vi "AutoDrive_sub.vi"(10 "Drive Control":T2={"Left X"=0, "Left Y"=0, "Right X"=0, "Power (100)"=100, "Wait (ms)"=100} {"Power (100)" min=-100 max=100}, 11 "NXT/EV3":T1) -> (3 "NXT/EV3 out":T1)   [LabVIEW 2012, in "Mecanum Drive.lvrbt"]
uses:
  Mecanum Drive.lvrbt
  SubVIs/auto_drive_TYP.ctl
  <vilib>/NXT/Subs/LVHSConnector.ctl
  <vilib>/NXT/LegoClasses/BrickReference/BrickReference.lvclass
  <vilib>/FTC/FTC ControllerState.ctl
  <vilib>/FTC/FTC POVState.ctl
  <vilib>/NXT/Hardware/Plugins/Tetrix DC Motor/TetrixDCMotorAddress.ctl
  <vilib>/NXT/Dual Mode Library/Display/drawNumber.vi
  <vilib>/NXT/NXTIO Xnodes/NXTIONodeSubVIs/TETRIX IO Move DC Motors.vi
  <vilib>/NXT/Dual Mode Library/Waits/Wait_Num(msec).vi
  <vilib>/NXT/NXTIO Xnodes/AddressXNode/NXTIOAddress.xnode
  <vilib>/NXT/NXTIO Xnodes/NXTIOXNode/NXTIO.xnode
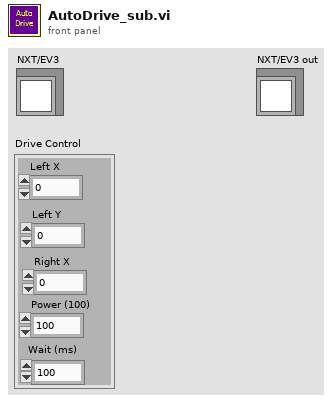
[diagram p1: front panel]
types:
  T1 = typedef "LVHSConnector.ctl" = refnum<class "BrickReference.lvclass">
  T2 = typedef "auto_drive_TYP.ctl" = cluster{"Left X":i8, "Left Y":i8, "Right X":i8, "Power (100)":i8, "Wait (ms)":u32}
  T3 = typedef "FTC ControllerState.ctl" = cluster{"Left X":i8, "Left Y":i8, "Right X":i8, "Right Y":i8, "Button Encoding 9-12":u8, "Button Encoding 1-8":u8, "POV":T4}
  T4 = typedef "FTC POVState.ctl" = i8
  T5 = typedef "TetrixDCMotorAddress.ctl" = i32
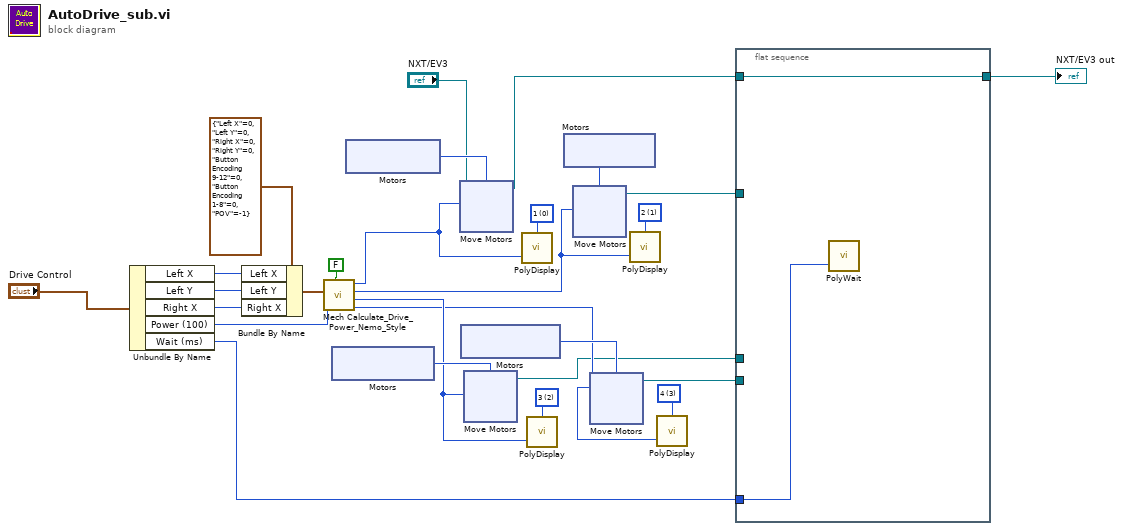
[diagram p0: block diagram]
diagram:
  w17 = i16 3 items=["1", "2", "3", "4", "5", "6", "7", "8", "9", "10", "11", "12"] ("Line")
  w19 = i16 2 items=["1", "2", "3", "4", "5", "6", "7", "8", "9", "10", "11", "12"] ("Line")
  w21 = i16 1 items=["1", "2", "3", "4", "5", "6", "7", "8", "9", "10", "11", "12"] ("Line")
  w22 = i16 0 items=["1", "2", "3", "4", "5", "6", "7", "8", "9", "10", "11", "12"] ("Line")
  n1 = Unbundle By Name("Drive Control") -> ("Left X"=w10:i8, "Left Y"=w9:i8, "Right X"=w8:i8, "Power (100)"=w2:i8, "Wait (ms)"=w1:u32)
  n2 = Bundle By Name(cluster=T3 {"Left X"=0, "Left Y"=0, "Right X"=0, "Right Y"=0, "Button Encoding 9-12"=0, "Button Encoding 1-8"=0, "POV"=-1} ("Controller State"), "Left X"=w10, "Left Y"=w9, "Right X"=w8) -> (w14:T3)
  n3 = call "Mech Calculate_Drive_Power_Nemo_Style.vi"("Reverse"=FALSE, "Controller State"=w14, "Power Level (100)"=w2) -> ("Right Rear Power"=w16:i8, "Right Front Power"=w18:i8, "Left Rear Power"=w20:i8, "Left Front Power"=w15:i8)  [unwired: 5 in]
  n4 = xnode ("Motors")() -> ("Motor"=w27:T5)
  n5 = xnode ("Motors")() -> ("Motor"=w24:T5)
  n6 = xnode ("Move Motors")("Power/Speed 1"=w15, "Motors"=w24, "NXT/EV3"="NXT/EV3") -> ("NXT/EV3"=w7:T1)
  n7 = xnode ("Motors")() -> ("Motor"=w26:T5)
  n8 = xnode ("Move Motors")("Power/Speed 1"=w18, "Motors"=w27) -> ("NXT/EV3"=w3:T1)  [unwired: 1 in]
  n9 = call-poly <vilib>:"PolyDisplay.vi"("number"=w15, "Line"=w22) -> ()  [unwired: 2 in, 1 out]
  n10 = call-poly <vilib>:"PolyDisplay.vi"("number"=w18, "Line"=w19) -> ()  [unwired: 2 in, 1 out]
  n11 = xnode ("Motors")() -> ("Motor"=w25:T5)
  n12 = xnode ("Move Motors")("Power/Speed 1"=w20, "Motors"=w25) -> ("NXT/EV3"=w5:T1)  [unwired: 1 in]
  n13 = xnode ("Move Motors")("Power/Speed 1"=w16, "Motors"=w26) -> ("NXT/EV3"=w4:T1)  [unwired: 1 in]
  n14 = call-poly <vilib>:"PolyDisplay.vi"("number"=w20, "Line"=w21) -> ()  [unwired: 2 in, 1 out]
  n15 = call-poly <vilib>:"PolyDisplay.vi"("number"=w16, "Line"=w17) -> ()  [unwired: 2 in, 1 out]
  n16 = flat-sequence {
    tunnel: w7 -> [w29]
    tunnel: [w29] -> w6
    tunnel: w5 -> [_]
    tunnel: w4 -> [_]
    tunnel: w3 -> [_]
    tunnel: w1 -> [w28]
    frame #0 {
      n17 = call-poly <vilib>:"PolyWait.vi"("Time (100 msec)"=w28) -> ()  [unwired: 3 in, 1 out]
    }
  }
  "NXT/EV3 out" <- w6
